vi "Uninit.vi"(11 "DAQ AI in":refnum<class "DAQ AI.lvclass">) -> (3 "DAQ AI out":refnum<class "DAQ AI.lvclass">)   [LabVIEW 2020, in "DAQ AI.lvlib" / "DAQ AI.lvclass"]
doc: "This method is the inverse of the Pre Launch Init.vi. This method is called unconditionally at the end of an actor's lifetime, even if there was an error in Pre Launch Init.vi. Note that the self Enqueuer for the actor is already invalid by the time this VI executes: within this method, the actor may send messages to its caller but not to itself. This method executes before Last Ack is sent.\n\nThis method neither receives nor produces an error cluster. It is designed to provide an unconditional release of acquired resources. Any error raised during release is considered to be irrelevant to the actor's lifetime. If the actor truly needs to report some error status, it may send a message to caller or include information within itself that callers can examine when handling Last Ack."
uses:
  DAQ AI.lvclass
  DAQ AI.lvclass/DAQ AI.ctl
  <vilib>/ActorFramework/Actor/Actor.lvclass
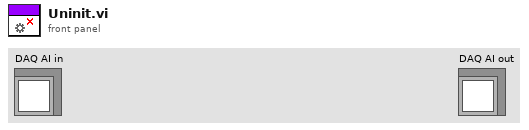
[diagram p1: front panel]
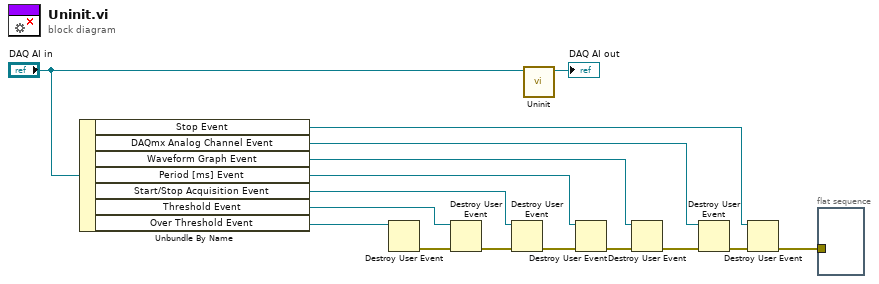
[diagram p0: block diagram]
diagram:
  n1 = Unbundle By Name("DAQ AI in") -> ("Stop Event"=w1:refnum<user-event>, "DAQmx Analog Channel Event"=w10:refnum<user-event>, "Waveform Graph Event"=w9:refnum<user-event>, "Period [ms] Event"=w8:refnum<user-event>, "Start/Stop Acquisition Event"=w7:refnum<user-event>, "Threshold Event"=w6:refnum<user-event>, "Over Threshold Event"=w5:refnum<user-event>)
  n2 = Destroy User Event(user event=w5) -> (error out=w4:errorcluster)  [unwired: 1 in]
  n3 = Destroy User Event(user event=w6, error in=w4) -> (error out=w15:errorcluster)
  n4 = Destroy User Event(user event=w7, error in=w15) -> (error out=w14:errorcluster)
  n5 = call-parent "Uninit.vi"("Actor in"="DAQ AI in") -> ("Actor out"=→"DAQ AI out":refnum<class "DAQ AI.lvclass">)  [unwired: 10 in]
  n6 = Destroy User Event(user event=w8, error in=w14) -> (error out=w13:errorcluster)
  n7 = Destroy User Event(user event=w9, error in=w13) -> (error out=w12:errorcluster)
  n8 = Destroy User Event(user event=w10, error in=w12) -> (error out=w3:errorcluster)
  n9 = Destroy User Event(user event=w1, error in=w3) -> (error out=w2:errorcluster)
  n10 = flat-sequence {
    tunnel: w2 -> [_]
    frame #0 {
    }
  }
